vi "read 4bytes(SubVI).vi"() -> (1 "Raw Z axis":i16, 2 "Raw Y axis":i16, 3 "Raw X axis":i16)   [LabVIEW 2019]
panel:
  out "SDA MAK 6":bool
  out "MAK6":bool
  out "high z axis":u8 format="%x"
  out "SDA MAK5":bool
  out "MAK5":bool
  out "low z axis":u8 format="%x"
  out "SDA MAK4":bool
  out "MAK4":bool
  out "high y axis":u8 format="%x"
  out "SDA MAK3":bool
  out "MAK3":bool
  out "low y axis":u8 format="%x"
  out "SDA MAK2":bool
  out "MAK2":bool
  out "High X axis":u8 format="%x"
  out "SDA MAK1":bool
  out "MAK1":bool
  out "low X axis  2":u8 format="%x"
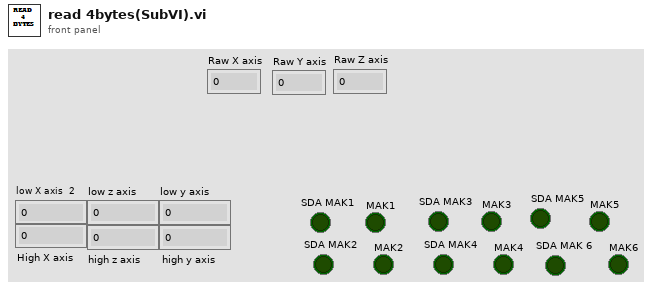
[diagram p1: front panel]
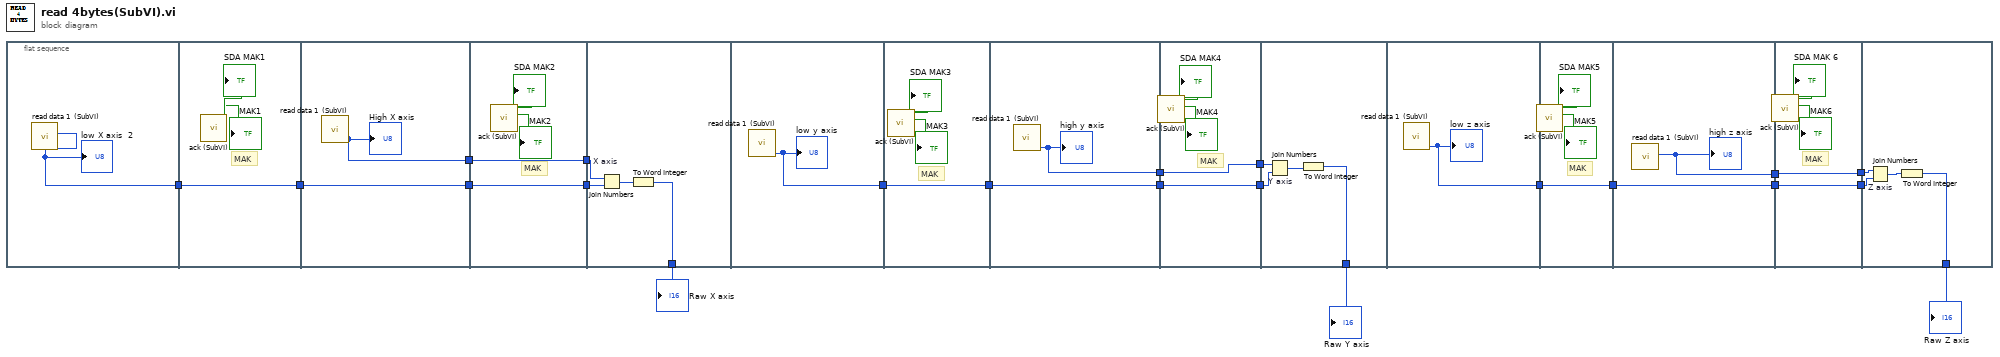
[diagram p0: block diagram]
diagram:
  n1 = flat-sequence {
    tunnel: [w22] -> w21
    tunnel: [w23] -> w20
    tunnel: w21 -> [w23]
    tunnel: w20 -> [w27]
    tunnel: [w27] -> w19
    tunnel: [w26] -> w18
    tunnel: w19 -> [w29]
    tunnel: w18 -> [w28]
    tunnel: [w29] -> w17
    tunnel: [w28] -> w16
    tunnel: w17 -> [w35]
    tunnel: w16 -> [w34]
    tunnel: [w32] -> w1
    tunnel: [w36] -> w15
    tunnel: w15 -> [w37]
    tunnel: [w37] -> w14
    tunnel: w14 -> [w41]
    tunnel: [w41] -> w13
    tunnel: [w40] -> w12
    tunnel: w13 -> [w43]
    tunnel: [w43] -> w11
    tunnel: w12 -> [w42]
    tunnel: [w42] -> w10
    tunnel: w11 -> [w49]
    tunnel: w10 -> [w48]
    tunnel: [w46] -> w2
    tunnel: [w50] -> w9
    tunnel: w9 -> [w51]
    tunnel: [w51] -> w8
    tunnel: [w55] -> w7
    tunnel: w8 -> [w54]
    tunnel: [w54] -> w6
    tunnel: w7 -> [w57]
    tunnel: [w57] -> w5
    tunnel: w6 -> [w56]
    tunnel: [w56] -> w4
    tunnel: w5 -> [w63]
    tunnel: w4 -> [w62]
    tunnel: [w60] -> w3
    frame #0 {
      n2 = call "read data 1  (SubVI).vi"() -> ("read data"=w22:u8)  [unwired: 10 in, 1 out]
      "low X axis  2" <- w22
    }
    frame #1 {
      # "MAK"
      n3 = call "ack (SubVI).vi"() -> ("ACK"=→"MAK1":bool, "SDA"=→"SDA MAK1":bool)  [unwired: 10 in]
    }
    frame #2 {
      n4 = call "read data 1  (SubVI).vi"() -> ("read data"=w26:u8)  [unwired: 10 in, 1 out]
      "High X axis" <- w26
    }
    frame #3 {
      # "MAK"
      n5 = call "ack (SubVI).vi"() -> ("ACK"=→"MAK2":bool, "SDA"=→"SDA MAK2":bool)  [unwired: 10 in]
    }
    frame #4 {
      n6 = Join Numbers "X axis"(hi=w34, lo=w35) -> ((hi.lo)=w33:u16)
      n7 = To Word Integer(number=w33) -> (16bit integer=w32:i16)
    }
    frame #5 {
      n8 = call "read data 1  (SubVI).vi"() -> ("read data"=w36:u8)  [unwired: 10 in, 1 out]
      "low y axis" <- w36
    }
    frame #6 {
      # "MAK"
      n9 = call "ack (SubVI).vi"() -> ("ACK"=→"MAK3":bool, "SDA"=→"SDA MAK3":bool)  [unwired: 10 in]
    }
    frame #7 {
      n10 = call "read data 1  (SubVI).vi"() -> ("read data"=w40:u8)  [unwired: 10 in, 1 out]
      "high y axis" <- w40
    }
    frame #8 {
      # "MAK"
      n11 = call "ack (SubVI).vi"() -> ("ACK"=→"MAK4":bool, "SDA"=→"SDA MAK4":bool)  [unwired: 10 in]
    }
    frame #9 {
      n12 = Join Numbers "Y axis"(hi=w48, lo=w49) -> ((hi.lo)=w47:u16)
      n13 = To Word Integer(number=w47) -> (16bit integer=w46:i16)
    }
    frame #10 {
      n14 = call "read data 1  (SubVI).vi"() -> ("read data"=w50:u8)  [unwired: 10 in, 1 out]
      "low z axis" <- w50
    }
    frame #11 {
      # "MAK"
      n15 = call "ack (SubVI).vi"() -> ("ACK"=→"MAK5":bool, "SDA"=→"SDA MAK5":bool)  [unwired: 10 in]
    }
    frame #12 {
      n16 = call "read data 1  (SubVI).vi"() -> ("read data"=w55:u8)  [unwired: 10 in, 1 out]
      "high z axis" <- w55
    }
    frame #13 {
      # "MAK"
      n17 = call "ack (SubVI).vi"() -> ("ACK"=→"MAK6":bool, "SDA"=→"SDA MAK 6":bool)  [unwired: 10 in]
    }
    frame #14 {
      n18 = Join Numbers "Z axis"(hi=w63, lo=w62) -> ((hi.lo)=w61:u16)
      n19 = To Word Integer(number=w61) -> (16bit integer=w60:i16)
    }
  }
  "Raw Z axis" <- w3
  "Raw Y axis" <- w2
  "Raw X axis" <- w1
